vi "Zero Coords.vi"(10 "Absolute Data":T1) -> (2 "Relative Data":T1)   [LabVIEW 2018, in "Stage Actor.lvlib"]
uses:
  Stage Actor.lvlib
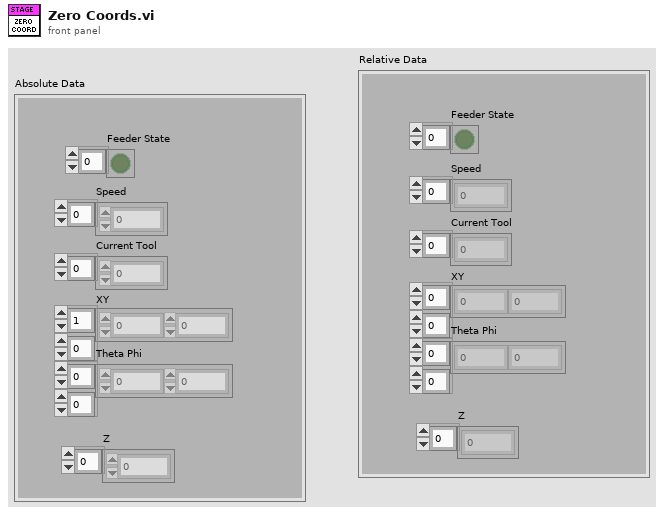
[diagram p1: front panel]
types:
  T1 = cluster{"XY":dbl[][], "Theta Phi":dbl[][], "Current Tool":i16[], "Speed":dbl[], "Feeder State":bool[], "Z":dbl[]}
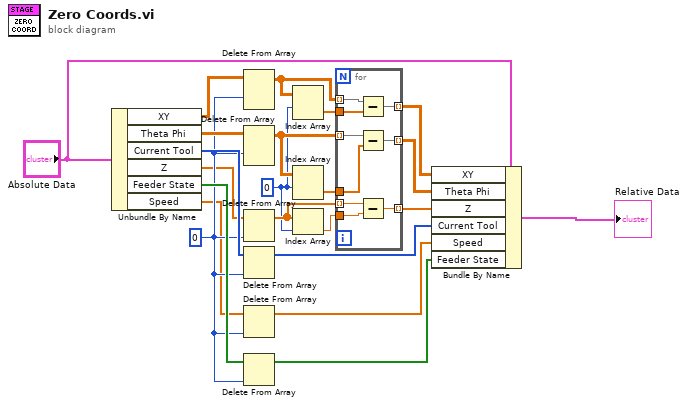
[diagram p0: block diagram]
diagram:
  w11 = 0
  w18 = 0
  n1 = Unbundle By Name("Absolute Data") -> ("XY"=w22:dbl[][], "Theta Phi"=w21:dbl[][], "Current Tool"=w20:i16[], "Z"=w2:dbl[], "Feeder State"=w19:bool[], "Speed"=w1:dbl[])
  n2 = Delete From Array(array=w22, index (row)=w18) -> (array with subset deleted=w14:dbl[][])  [unwired: 2 in, 1 out]
  n3 = Delete From Array(array=w21, index (row)=w18) -> (array with subset deleted=w12:dbl[][])  [unwired: 2 in, 1 out]
  n4 = Delete From Array(array=w2, index=w18) -> (array with subset deleted=w13:dbl[])  [unwired: 1 in, 1 out]
  n5 = Delete From Array(array=w20, index=w18) -> (array with subset deleted=w6:i16[])  [unwired: 1 in, 1 out]
  n6 = Delete From Array(array=w1, index=w18) -> (array with subset deleted=w5:dbl[])  [unwired: 1 in, 1 out]
  n7 = Delete From Array(array=w19, index=w18) -> (array with subset deleted=w4:bool[])  [unwired: 1 in, 1 out]
  n8 = Index Array(array=w14, index (row)=w11) -> (element=w17:dbl[])  [unwired: 1 in]
  n9 = Index Array(array=w12, index (row)=w11) -> (element=w16:dbl[])  [unwired: 1 in]
  n10 = Index Array(array=w13, index=w11) -> (element=w15:dbl)
  n11 = for {
    tunnel: w17 -> [w30]
    tunnel: w16 -> [w27]
    tunnel: w15 -> [w25]
    tunnel: w14 -> [w31] mode=indexing
    tunnel: w13 -> [w26] mode=indexing
    tunnel: w12 -> [w28] mode=indexing
    tunnel: [w29] -> w9 mode=indexing
    tunnel: [w24] -> w7 mode=indexing
    tunnel: [w23] -> w8 mode=indexing
    n12 = Subtract(x=w31, y=w30) -> (x-y=w29:dbl[])
    n13 = Subtract(x=w28, y=w27) -> (x-y=w23:dbl[])
    n14 = Subtract(x=w26, y=w25) -> (x-y=w24:dbl)
  }
  n15 = Bundle By Name(cluster="Absolute Data", "XY"=w9, "Theta Phi"=w8, "Z"=w7, "Current Tool"=w6, "Speed"=w5, "Feeder State"=w4) -> (→"Relative Data":T1)
